vi "HVSM_CmdStr.vi"(1 "HVSM":T1 {"司机座椅加热状态" items=["关闭", "Level1", "Level2", "Level3", "预留", "错误"]; "副驾座椅加热状态" items=["关闭", "Level1", "Level2", "Level3", "预留", "错误"]}) -> (0 "CmdStr":string)   [LabVIEW 2013]
uses:
  HVSM.ctl
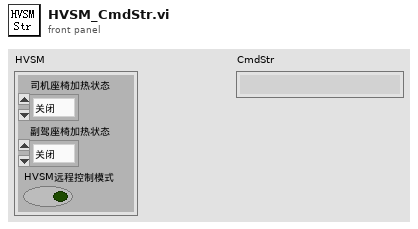
[diagram p1: front panel]
types:
  T1 = typedef "HVSM.ctl" = cluster{"司机座椅加热状态":u8, "副驾座椅加热状态":u8, "HVSM远程控制模式":bool}
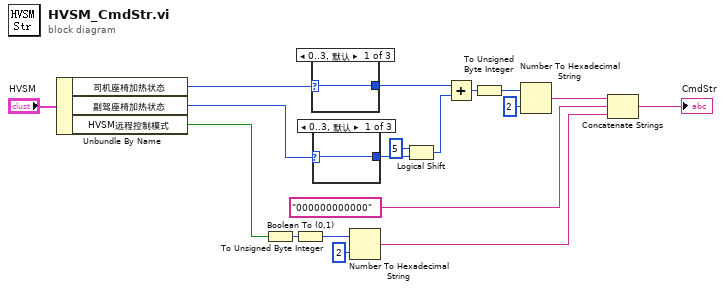
[diagram p0: block diagram]
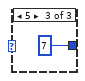
[diagram p3: hidden frame]
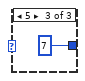
[diagram p5: hidden frame]
diagram:
  n1 = Unbundle By Name("HVSM") -> ("司机座椅加热状态"=w3:u8, "副驾座椅加热状态"=w2:u8, "HVSM远程控制模式"=w1:bool)
  n2 = Boolean To (0,1)(Boolean=w1) -> (0, 1=w14:i16)
  n3 = To Unsigned Byte Integer(number=w14) -> (unsigned 8bit integer=w7:u8)
  n4 = case shown="0..3, 默认" w3 {
    selector: w3 -> [w19 w20 _]
    tunnel: [w19 w20 u8 7] -> w16
    frame 0..3, Default {
    }
    frame 4 {
    }
    frame 5 {
    }
  }
  n5 = case shown="0..3, 默认" w2 {
    selector: w2 -> [w22 w23 _]
    tunnel: [w22 w23 u8 7] -> w18
    frame 0..3, Default {
    }
    frame 4 {
    }
    frame 5 {
    }
  }
  n6 = Number To Hexadecimal String(1:i16 2 ("宽度(-)"), 2:w7) -> (0:w6:string)
  n7 = Logical Shift(y=i16 5, x=w18) -> (x << y=w15:u8)
  n8 = Add(x=w16, y=w15) -> (x+y=w13:u8)
  n9 = To Unsigned Byte Integer(number=w13) -> (unsigned 8bit integer=w12:u8)
  n10 = Number To Hexadecimal String(1:i16 2 ("宽度(-)"), 2:w12) -> (0:w10:string)
  n11 = Concatenate Strings(w10, "000000000000", w6) -> (→"CmdStr":string)
